vi "Read Measurement Statistics.vi"(0 "VISA resource name":refnum<visa-resource-name>, 11 "error in (no error)":errorcluster) -> (2 "Standard Deviation":dbl, 3 "Minimum Value":dbl, 4 "VISA resource name out":refnum<visa-resource-name>, 6 "Arithmetic Mean":dbl, 8 "Measurement Count":dbl, 10 "Maximum Value":dbl, 14 "Peak-to-peak Value":dbl, 15 "error out":errorcluster)   [LabVIEW 2020, in "Agilent 3446X Series.lvlib"]
doc: "Reads the measurement statistics."
uses:
  <instrlib>/Agilent 3446X Series/Agilent 3446X Series.lvlib
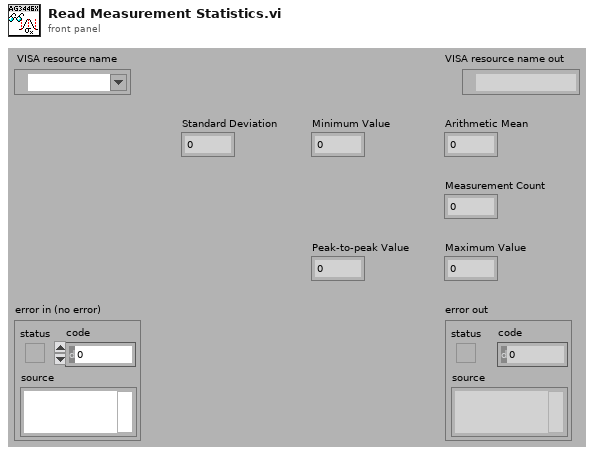
[diagram p1: front panel]
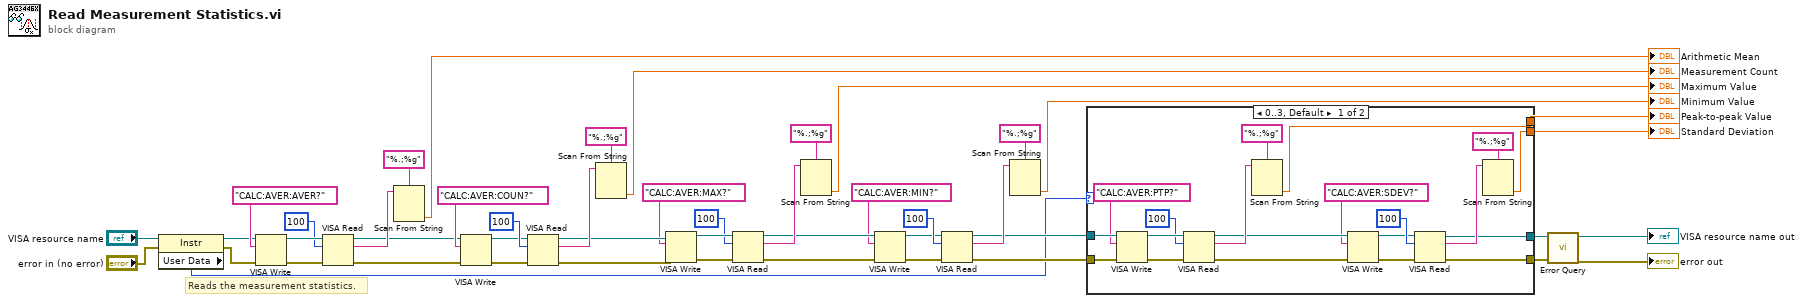
[diagram p0: block diagram]
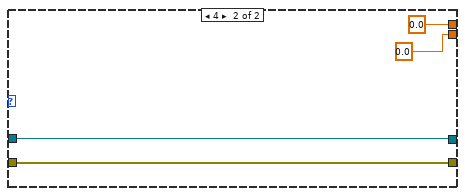
[diagram p2: hidden frame]
diagram:
  # "Reads the measurement statistics."
  n1 = property class="Instr"(reference="VISA resource name", error in="error in (no error)") -> (reference out=w4:refnum<visa-resource-name>, error out=w2:errorcluster, "User Data"=w1:u32)
  n2 = VISA Write(VISA resource name=w4, write buffer="CALC:AVER:AVER?", error in (no error)=w2) -> (VISA resource name out=w43:refnum<visa-resource-name>, error out=w44:errorcluster)  [unwired: 1 out]
  n3 = VISA Read(VISA resource name=w43, byte count=u32 100, error in (no error)=w44) -> (VISA resource name out=w34:refnum<visa-resource-name>, read buffer=w41:string, error out=w33:errorcluster)  [unwired: 1 out]
  n4 = Scan From String(format string="%.;%g", input string=w41) -> (output 1=→"Arithmetic Mean":dbl)  [unwired: 2 in, 4 out]
  n5 = VISA Write(VISA resource name=w34, write buffer="CALC:AVER:COUN?", error in (no error)=w33) -> (VISA resource name out=w36:refnum<visa-resource-name>, error out=w22:errorcluster)  [unwired: 1 out]
  n6 = VISA Read(VISA resource name=w36, byte count=u32 100, error in (no error)=w22) -> (VISA resource name out=w24:refnum<visa-resource-name>, read buffer=w38:string, error out=w23:errorcluster)  [unwired: 1 out]
  n7 = Scan From String(format string="%.;%g", input string=w38) -> (output 1=→"Measurement Count":dbl)  [unwired: 2 in, 4 out]
  n8 = VISA Write(VISA resource name=w24, write buffer="CALC:AVER:MAX?", error in (no error)=w23) -> (VISA resource name out=w32:refnum<visa-resource-name>, error out=w21:errorcluster)  [unwired: 1 out]
  n9 = VISA Read(VISA resource name=w32, byte count=u32 100, error in (no error)=w21) -> (VISA resource name out=w20:refnum<visa-resource-name>, read buffer=w30:string, error out=w19:errorcluster)  [unwired: 1 out]
  n10 = Scan From String(format string="%.;%g", input string=w30) -> (output 1=→"Maximum Value":dbl)  [unwired: 2 in, 4 out]
  n11 = VISA Write(VISA resource name=w20, write buffer="CALC:AVER:MIN?", error in (no error)=w19) -> (VISA resource name out=w25:refnum<visa-resource-name>, error out=w18:errorcluster)  [unwired: 1 out]
  n12 = VISA Read(VISA resource name=w25, byte count=u32 100, error in (no error)=w18) -> (VISA resource name out=w16:refnum<visa-resource-name>, read buffer=w27:string, error out=w17:errorcluster)  [unwired: 1 out]
  n13 = Scan From String(format string="%.;%g", input string=w27) -> (output 1=→"Minimum Value":dbl)  [unwired: 2 in, 4 out]
  n14 = case shown="0..3, Default" w1 {
    tunnel: w17 -> [w59 w70]
    tunnel: w16 -> [w58 w71]
    tunnel: [w53 w71] -> w15
    tunnel: [w52 w70] -> w14
    tunnel: [w51 0.0] -> w13
    tunnel: [w50 0.0] -> w12
    frame 0..3, Default {
      n15 = VISA Write(VISA resource name=w58, write buffer="CALC:AVER:PTP?", error in (no error)=w59) -> (VISA resource name out=w67:refnum<visa-resource-name>, error out=w57:errorcluster)  [unwired: 1 out]
      n16 = VISA Read(VISA resource name=w67, byte count=u32 100, error in (no error)=w57) -> (VISA resource name out=w56:refnum<visa-resource-name>, read buffer=w65:string, error out=w55:errorcluster)  [unwired: 1 out]
      n17 = Scan From String(format string="%.;%g", input string=w65) -> (output 1=w50:dbl)  [unwired: 2 in, 4 out]
      n18 = VISA Write(VISA resource name=w56, write buffer="CALC:AVER:SDEV?", error in (no error)=w55) -> (VISA resource name out=w60:refnum<visa-resource-name>, error out=w54:errorcluster)  [unwired: 1 out]
      n19 = VISA Read(VISA resource name=w60, byte count=u32 100, error in (no error)=w54) -> (VISA resource name out=w53:refnum<visa-resource-name>, read buffer=w62:string, error out=w52:errorcluster)  [unwired: 1 out]
      n20 = Scan From String(format string="%.;%g", input string=w62) -> (output 1=w51:dbl)  [unwired: 2 in, 4 out]
    }
    frame 4 {
    }
  }
  "Peak-to-peak Value" <- w12
  "Standard Deviation" <- w13
  n21 = call <instrlib>:"Error Query.vi"("error in (no error)"=w14, "VISA resource name"=w15) -> ("error out"=→"error out":errorcluster, "VISA resource name out"=→"VISA resource name out":refnum<visa-resource-name>)  [unwired: 8 out]
